vi "Get Query String.vi"(8 "error in (no error)":errorcluster, 9 "HTML Entity (F)":bool, 11 "URI-Component.Path in":refnum<class "URI-Component.Query.lvclass">) -> (0 "error out":errorcluster, 2 "query-component":string, 3 "URI-Component.Path out":refnum<class "URI-Component.Query.lvclass">)   [LabVIEW 2013, in "openURI.lvlib" / "URI-Component.Query.lvclass"]
uses:
  URI-Component.Query.lvclass
  URI-Component.Query.lvclass/URI-Component.Query.ctl
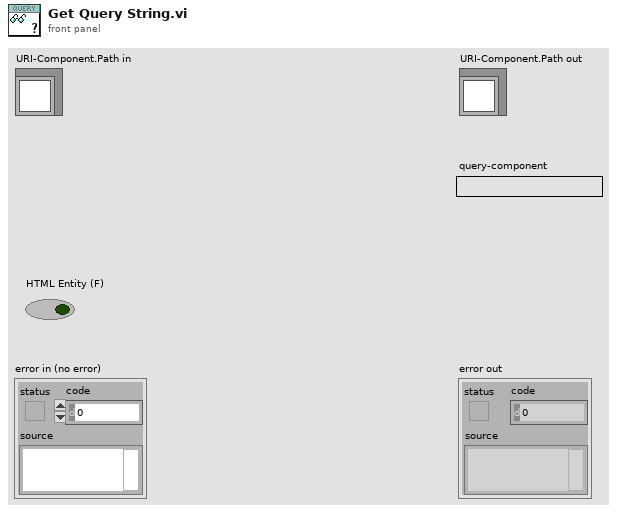
[diagram p1: front panel]
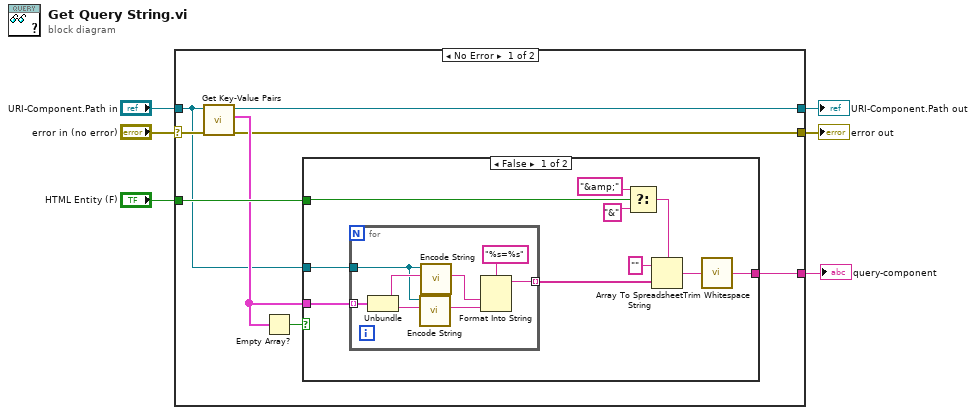
[diagram p0: block diagram]
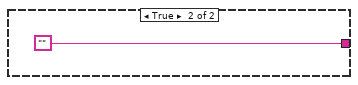
[diagram p2: hidden frame]
diagram:
  n1 = case shown="No Error" "error in (no error)" {
    selector: "error in (no error)" -> [w9 w35]
    tunnel: [w8 w35] -> w5
    tunnel: [w14 w34] -> w3
    tunnel: "URI-Component.Path in" -> [w7 w34]
    tunnel: [w10 _] -> w2
    tunnel: "HTML Entity (F)" -> [w12 _]
    frame No Error {
      n2 = call "Get Key-Value Pairs.vi"("error in (no error)"=w9, "URI-Component.Query in"=w7) -> ("error out"=w8:errorcluster, "Query"=w11:cluster{"argument":string, "value":string}[], "URI-Component.Query"=w14:refnum<class "URI-Component.Query.lvclass">)  [unwired: 7 in]
      n3 = Empty Array?(array=w11) -> (empty?=w13:bool)
      n4 = case shown="False" w13 {
        tunnel: w11 -> [w24 _]
        tunnel: [w20 ""] -> w10
        tunnel: w12 -> [w19 _]
        tunnel: w7 -> [w15 _]
        frame False {
          n5 = for {
            tunnel: w24 -> [w32] mode=indexing
            tunnel: [w30] -> w23 mode=indexing
            tunnel: w15 -> [w25]
            n6 = Unbundle(w32) -> ("argument"=w29:string, "value"=w26:string)
            n7 = call-dynamic "Encode String.vi"("String"=w26, "URI-Component.Query"=w25) -> ("Encoded String"=w27:string)  [unwired: 9 in]
            n8 = call-dynamic "Encode String.vi"("String"=w29, "URI-Component.Query"=w25) -> ("Encoded String"=w28:string)  [unwired: 9 in]
            n9 = Format Into String(format string="%s=%s", w28, w27) -> (resulting string=w30:string)  [unwired: 2 in, 1 out]
          }
          n10 = Select(t="&amp;" ("delimiter (Tab)"), s=w19, f="&" ("delimiter (Tab)")) -> (s? t:f=w18:string)
          n11 = Array To Spreadsheet String(delimiter (Tab)=w18, array=w23, 3:"" ("format string")) -> (spreadsheet string=w21:string)
          n12 = call <vilib>:"Trim Whitespace.vi"("string"=w21) -> ("trimmed string"=w20:string)  [unwired: 1 in]
        }
        frame True {
        }
      }
    }
    frame Error {
    }
  }
  "error out" <- w5
  "URI-Component.Path out" <- w3
  "query-component" <- w2
